vi "test_libssh2_userauth_list.vi"() -> ()   [LabVIEW 2013, in "libssh2_integration_tests.lvlib"]
uses:
  libssh2_integration_tests.lvlib
  libssh2/libssh2_init_default.vi
  libssh2/libssh2_session_handshake_tcp.vi
  libssh2/libssh2.lvlib
  <vilib>/addons/_JKI Toolkits/Caraya/classes/Test/Test.lvclass
  support/support.lvlib
  <vilib>/addons/_JKI Toolkits/Caraya/classes/Assert/Assert.lvclass
panel:
  out "error out":errorcluster
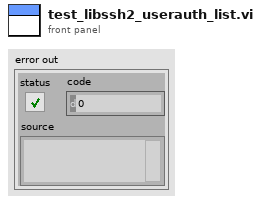
[diagram p1: front panel]
types:
  T1 = typedef "libssh2.lvlib/Session Refnum.ctl" = refnum<k1>
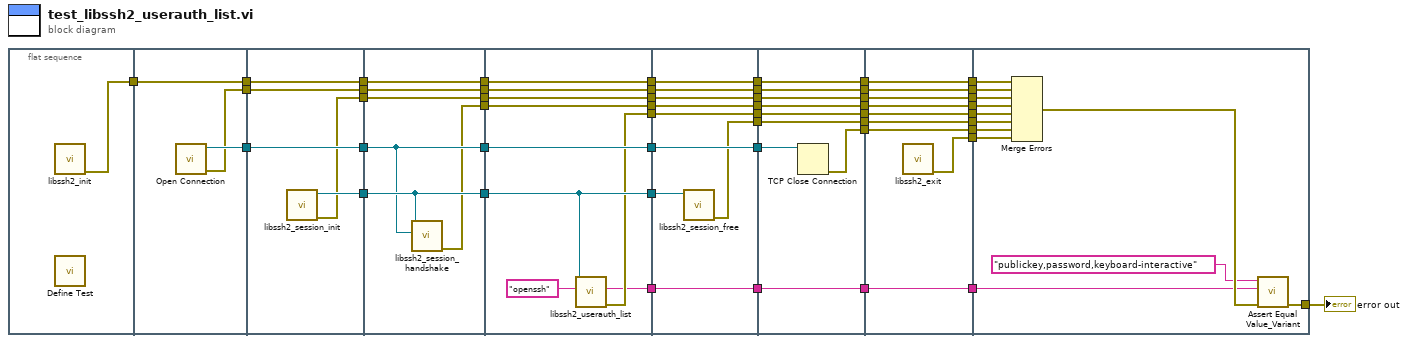
[diagram p0: block diagram]
diagram:
  n1 = flat-sequence {
    tunnel: [w50] -> w49
    tunnel: [w53] -> w48
    tunnel: w49 -> [w52]
    tunnel: [w52] -> w47
    tunnel: [w51] -> w46
    tunnel: w48 -> [w58]
    tunnel: [w58] -> w16
    tunnel: w47 -> [w57]
    tunnel: [w57] -> w15
    tunnel: w46 -> [w56]
    tunnel: [w56] -> w14
    tunnel: [w55] -> w13
    tunnel: [w54] -> w12
    tunnel: w16 -> [w60]
    tunnel: [w60] -> w34
    tunnel: w15 -> [w64]
    tunnel: [w64] -> w33
    tunnel: w14 -> [w63]
    tunnel: [w63] -> w32
    tunnel: [w62] -> w31
    tunnel: w13 -> [w62]
    tunnel: w12 -> [w61]
    tunnel: [w61] -> w30
    tunnel: [w59] -> w29
    tunnel: w34 -> [w73]
    tunnel: [w73] -> w8
    tunnel: w33 -> [w72]
    tunnel: [w72] -> w7
    tunnel: w32 -> [w71]
    tunnel: [w71] -> w6
    tunnel: w31 -> [w68]
    tunnel: w30 -> [w70]
    tunnel: [w70] -> w5
    tunnel: w29 -> [w69]
    tunnel: [w69] -> w4
    tunnel: [w67] -> w3
    tunnel: [w68] -> w2
    tunnel: [w65] -> w1
    tunnel: w8 -> [w82]
    tunnel: [w82] -> w26
    tunnel: w7 -> [w81]
    tunnel: [w81] -> w25
    tunnel: w6 -> [w80]
    tunnel: [w80] -> w24
    tunnel: w5 -> [w79]
    tunnel: [w79] -> w23
    tunnel: w4 -> [w78]
    tunnel: [w78] -> w22
    tunnel: w3 -> [w77]
    tunnel: [w77] -> w21
    tunnel: [w76] -> w18
    tunnel: [w75] -> w9
    tunnel: w1 -> [w75]
    tunnel: w2 -> [w74]
    tunnel: w26 -> [w91]
    tunnel: w25 -> [w90]
    tunnel: [w90] -> w45
    tunnel: w24 -> [w89]
    tunnel: [w89] -> w44
    tunnel: [w88] -> w43
    tunnel: w23 -> [w87]
    tunnel: [w87] -> w42
    tunnel: w22 -> [w86]
    tunnel: [w86] -> w41
    tunnel: w21 -> [w85]
    tunnel: [w85] -> w28
    tunnel: [w84] -> w19
    tunnel: w18 -> [w84]
    tunnel: [w83] -> w10
    tunnel: w9 -> [w83]
    tunnel: w45 -> [w100]
    tunnel: [w100] -> w40
    tunnel: w44 -> [w99]
    tunnel: [w99] -> w39
    tunnel: w43 -> [w98]
    tunnel: [w98] -> w38
    tunnel: [w97] -> w37
    tunnel: w42 -> [w96]
    tunnel: [w96] -> w36
    tunnel: w41 -> [w95]
    tunnel: [w95] -> w35
    tunnel: w28 -> [w94]
    tunnel: [w94] -> w27
    tunnel: [w93] -> w20
    tunnel: w19 -> [w93]
    tunnel: [w92] -> w11
    tunnel: w10 -> [w92]
    tunnel: w40 -> [w112]
    tunnel: w39 -> [w111]
    tunnel: w38 -> [w110]
    tunnel: w37 -> [w109]
    tunnel: w36 -> [w108]
    tunnel: [w106] -> w17
    tunnel: w35 -> [w105]
    tunnel: w27 -> [w104]
    tunnel: w20 -> [w103]
    tunnel: w11 -> [w102]
    frame #0 {
      n2 = call-poly "libssh2_init.vi"() -> ("error out"=w50:errorcluster)  [unwired: 11 in]
      n3 = call <vilib>:"Define Test.vi"() -> ()  [unwired: 10 in, 2 out]
    }
    frame #1 {
      n4 = call "Open Connection.vi"() -> ("error out"=w51:errorcluster, "connection ID"=w53:refnum<k5>)  [unwired: 10 in]
    }
    frame #2 {
      n5 = call "libssh2_session_init.vi"() -> ("error out"=w54:errorcluster, "session"=w55:T1)  [unwired: 10 in]
    }
    frame #3 {
      n6 = call-poly "libssh2_session_handshake.vi"("tcp connection"=w60, "session"=w62) -> ("error out"=w59:errorcluster)  [unwired: 9 in]
    }
    frame #4 {
      n7 = call "libssh2_userauth_list.vi"("username"="openssh", "session"=w68) -> ("error out"=w67:errorcluster, "supported authentication schemes"=w65:string)  [unwired: 8 in]
    }
    frame #5 {
      n8 = call "libssh2_session_free.vi"("session"=w74) -> ("error out"=w76:errorcluster)  [unwired: 10 in]
    }
    frame #6 {
      n9 = TCP Close Connection(connection ID=w91) -> (error out=w88:errorcluster)  [unwired: 2 in, 1 out]
    }
    frame #7 {
      n10 = call "libssh2_exit.vi"() -> ("error out"=w97:errorcluster)  [unwired: 11 in]
    }
    frame #8 {
      n11 = Merge Errors(w112, w111, w108, w105, w104, w103, w110, w109) -> (w107:errorcluster)
      n12 = call <vilib>:"Assert Equal Value_Variant.vi"("error in (no error)"=w107, "Y"=w102, "X"="publickey,password,keyboard-interactive" ("supported authentication schemes")) -> ("error out"=w106:errorcluster)  [unwired: 7 in, 1 out]
    }
  }
  "error out" <- w17
